vi "Serial Write Read.vi"(8 "error in (no error)":errorcluster, 9 "Delay Time (s)":dbl=1.0, 10 "write buffer":string, 11 "VISA resource name":refnum<visa-resource-name>) -> (0 "error out":errorcluster, 2 "read buffer":string, 3 "VISA resource name out":refnum<visa-resource-name>, 4 "read return count":u32, 5 "write return count":u32)   [LabVIEW 2025, in "SerialPort.lvlib"]
uses:
  <vilib>/Serial Port/SerialPort.lvlib
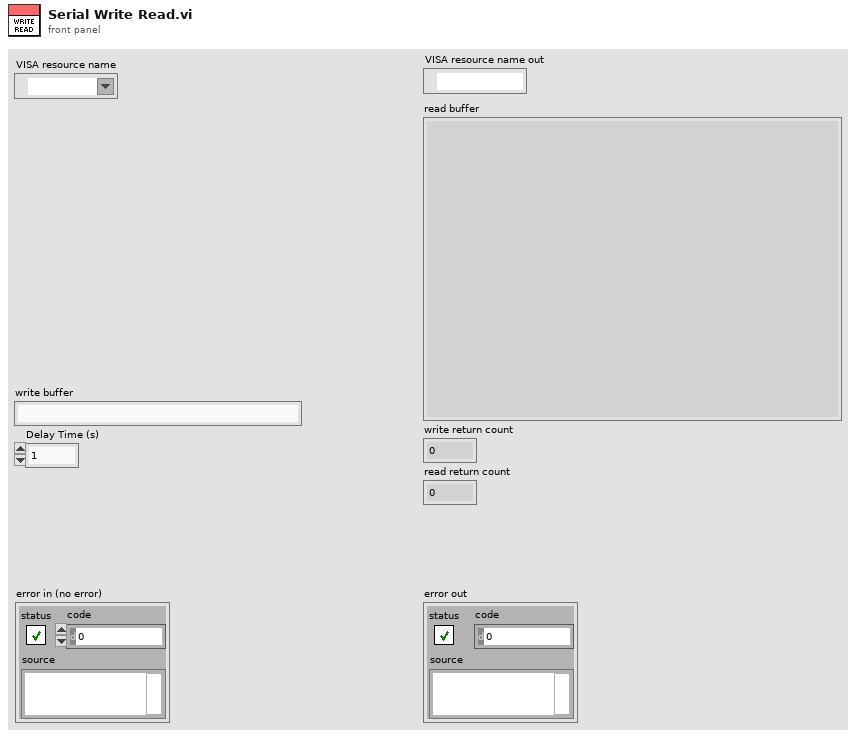
[diagram p1: front panel]
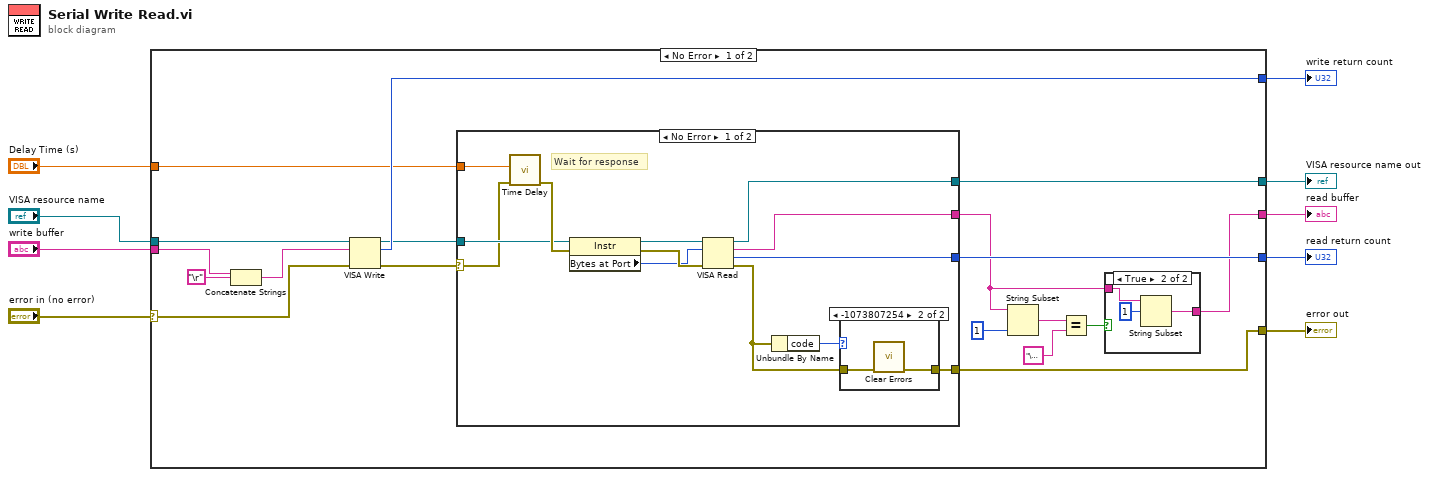
[diagram p0: block diagram]
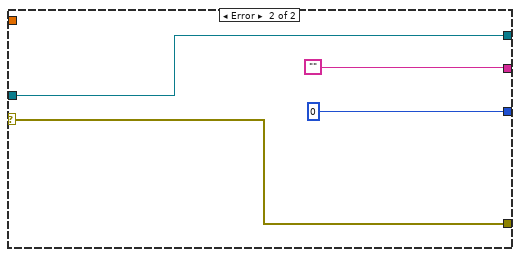
[diagram p4: hidden frame]
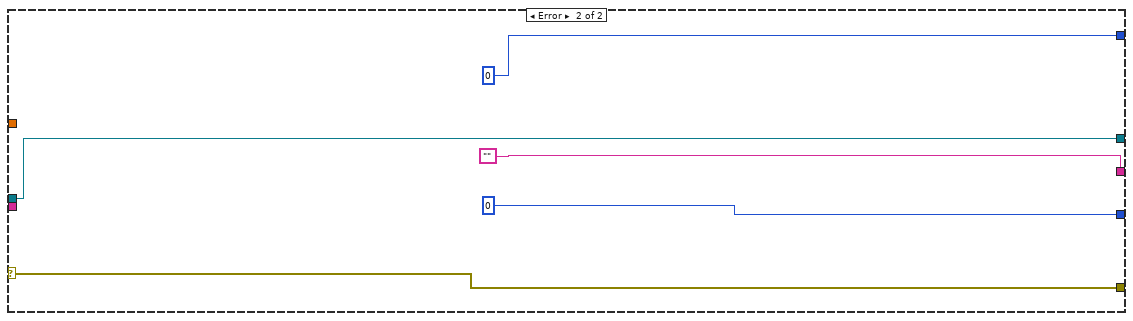
[diagram p5: hidden frame]
diagram:
  n1 = case shown="No Error" "error in (no error)" {
    selector: "error in (no error)" -> [w19 w53]
    tunnel: "VISA resource name" -> [w20 w56]
    tunnel: "write buffer" -> [w11 _]
    tunnel: [w27 u32 0 ("return count")] -> w8
    tunnel: "Delay Time (s)" -> [w26 _]
    tunnel: [w24 w56] -> w6
    tunnel: [w23 w53] -> w5
    tunnel: [w17 ""] -> w4
    tunnel: [w22 u32 0 ("return count")] -> w3
    frame No Error {
      n2 = Concatenate Strings(w11, "\r") -> (w10:string)
      n3 = VISA Write(VISA resource name=w20, write buffer=w10, error in (no error)=w19) -> (VISA resource name out=w25:refnum<visa-resource-name>, return count=w27:u32, error out=w21:errorcluster)
      n4 = case shown="No Error" w21 {
        selector: w21 -> [w35 w50]
        tunnel: w26 -> [w44 _]
        tunnel: w25 -> [w42 w51]
        tunnel: [w38 w51] -> w24
        tunnel: [w34 w50] -> w23
        tunnel: [w37 ""] -> w18
        tunnel: [w36 u32 0 ("return count")] -> w22
        frame No Error {
          # "Wait for response"
          n5 = call "Time Delay"("error in (no error)"=w35, "Delay Time (s)"=w44) -> ("error out"=w43:errorcluster)  [unwired: 9 in]
          n6 = property class="Instr"(reference=w42, error in=w43) -> (reference out=w41:refnum<visa-resource-name>, error out=w40:errorcluster, "Bytes at Port"=w39:u32)
          n7 = VISA Read(VISA resource name=w41, byte count=w39, error in (no error)=w40) -> (VISA resource name out=w38:refnum<visa-resource-name>, read buffer=w37:string, return count=w36:u32, error out=w33:errorcluster)
          n8 = Unbundle By Name(w33) -> ("code"=w32:i32)
          n9 = case shown="-1073807254" w32 {
            tunnel: w33 -> [w45 w47]
            tunnel: [w45 w46] -> w34
            frame Default {
            }
            frame -1073807254 {
              n10 = call <vilib>:"Clear Errors.vi"("error in (no error)"=w47) -> ("error out"=w46:errorcluster)  [unwired: 5 in, 1 out]
            }
          }
        }
        frame Error {
        }
      }
      n11 = String Subset(string=w18, length (rest)=1 ("offset (0)")) -> (substring=w16:string)  [unwired: 1 in]
      n12 = Equal?(x=w16, y="\u0000") -> (x = y?=w13:bool)
      n13 = case shown="True" w13 {
        tunnel: w18 -> [w28 w31]
        tunnel: [w28 w29] -> w17
        frame False {
        }
        frame True {
          n14 = String Subset(string=w31, offset (0)=1) -> (substring=w29:string)  [unwired: 1 in]
        }
      }
    }
    frame Error {
    }
  }
  "error out" <- w5
  "VISA resource name out" <- w6
  "write return count" <- w8
  "read buffer" <- w4
  "read return count" <- w3
